vi "puls_generator_control.VI"() -> ()   [LabVIEW 2015]
uses:
  board.vis/Globals.vi
panel:
  in  "TM0H":u16
  in  "TM0L":u16=1000
  in  "DO8":u16
  in  "TO8":u16
  in  "DO7":u16
  in  "TO7":u16
  in  "DO6":u16
  in  "TO6":u16
  in  "DO5":u16
  in  "TO5":u16
  in  "DO4":u16
  in  "T04":u16
  in  "DO3":u16
  in  "TO3":u16
  in  "D02":u16=100
  in  "TO2":u16=10
  in  "Send O CTRL":bool
  out "cams recognised":u8=2
  # "Tn: delay"
  # "Dn: duration"
  # "*5ns"
  # "TO1: T0 main clock"
  # "period"
  # "*10ns"
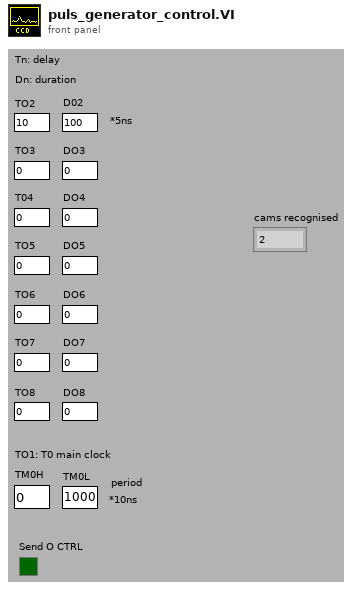
[diagram p1: front panel]
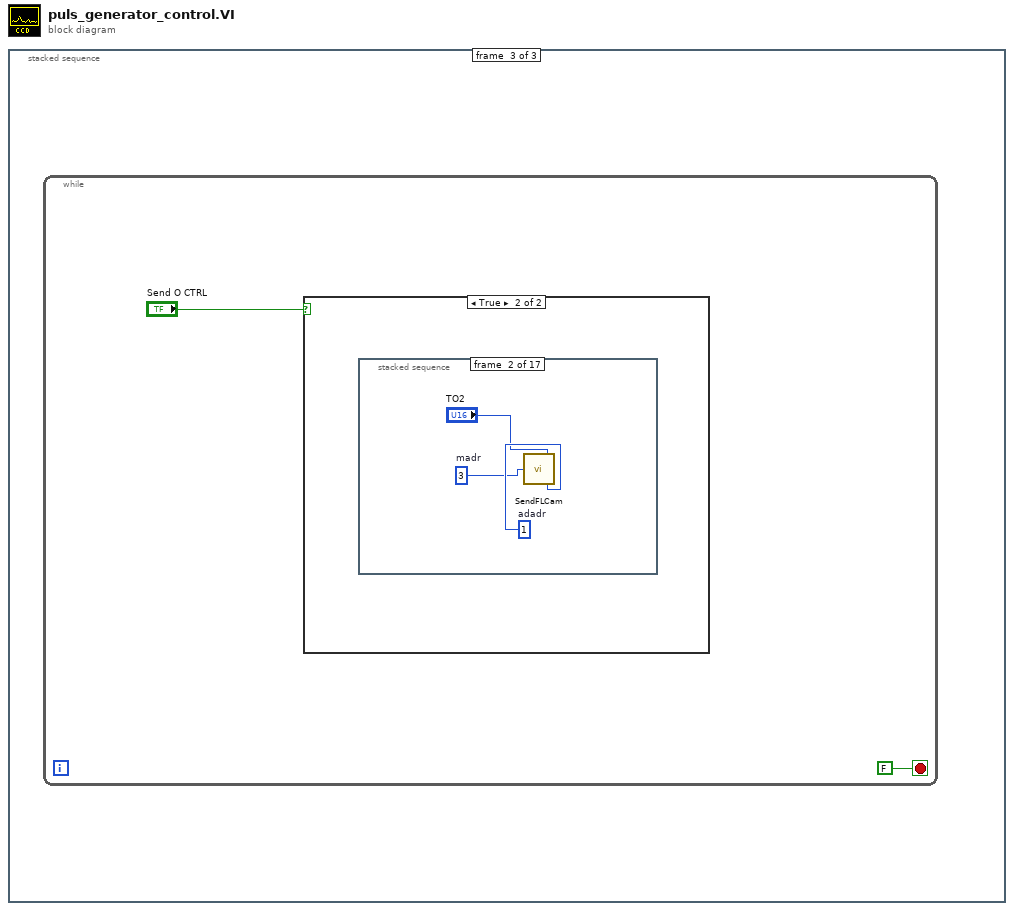
[diagram p0: block diagram]
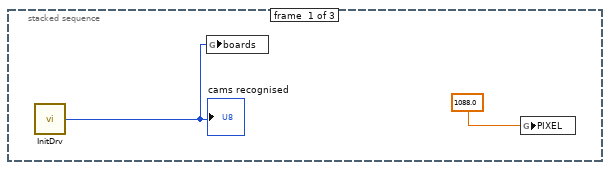
[diagram p2: hidden frame]
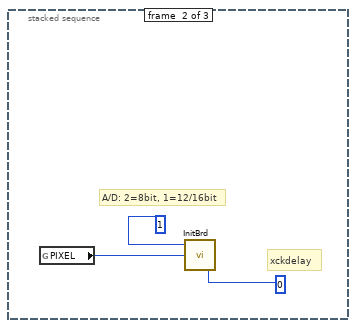
[diagram p3: hidden frame]
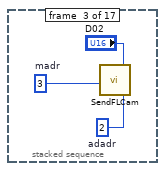
[diagram p6: hidden frame]
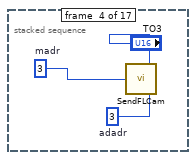
[diagram p7: hidden frame]
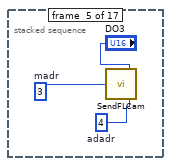
[diagram p8: hidden frame]
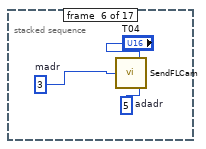
[diagram p9: hidden frame]
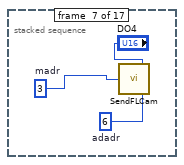
[diagram p10: hidden frame]
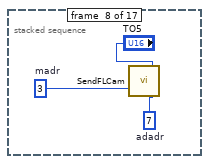
[diagram p11: hidden frame]
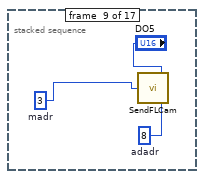
[diagram p12: hidden frame]
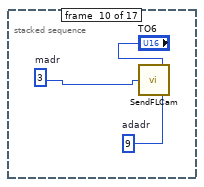
[diagram p13: hidden frame]
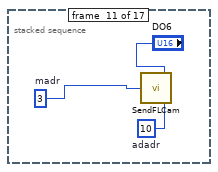
[diagram p14: hidden frame]
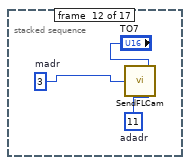
[diagram p15: hidden frame]
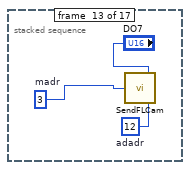
[diagram p16: hidden frame]
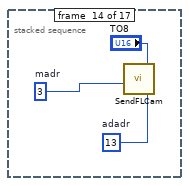
[diagram p17: hidden frame]
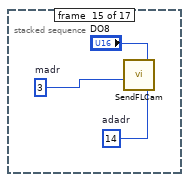
[diagram p18: hidden frame]
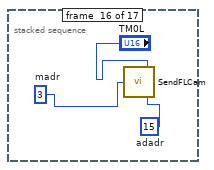
[diagram p19: hidden frame]
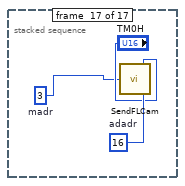
[diagram p20: hidden frame]
diagram:
  n1 = stacked-sequence {
    frame #0 {
      n2 = call "InitDrv.vi"() -> ("Boards"=w2:u8)  [unwired: 1 in]
      "cams recognised" <- w2
      n3 = global write "Globals.vi" "boards"(w2) -> ()
      n4 = global write "Globals.vi" "PIXEL"(1088.0) -> ()
    }
    frame #1 {
      # "xckdelay"
      # "A/D: 2=8bit, 1=12/16bit"
      n5 = global read "Globals.vi" "PIXEL"() -> (w3:u32)
      n6 = call "InitBrd.vi"("xckdly"=u32 0, "pixel"=w3, "flag816"=u32 1) -> ()  [unwired: 3 in]
    }
    frame #2 {
      n7 = while {
        stop <- FALSE stop-if-true
        n8 = case shown="True" "Send O CTRL" {
          frame False {
          }
          frame True {
            n9 = stacked-sequence {
              frame #0 {
              }
              frame #1 {
                w10 = 1  # adadr
                w9 = 3  # madr
                n10 = call "SendFLCam.vi"("madr"=w9, "data"="TO2", "adadr"=w10) -> ()
              }
              frame #2 {
                w12 = 2  # adadr
                w13 = 3  # madr
                n11 = call "SendFLCam.vi"("madr"=w13, "data"="D02", "adadr"=w12) -> ()
              }
              frame #3 {
                w16 = 3  # adadr
                w15 = 3  # madr
                n12 = call "SendFLCam.vi"("madr"=w15, "data"="TO3", "adadr"=w16) -> ()
              }
              frame #4 {
                w19 = 4  # adadr
                w18 = 3  # madr
                n13 = call "SendFLCam.vi"("madr"=w18, "data"="DO3", "adadr"=w19) -> ()
              }
              frame #5 {
                w22 = 5  # adadr
                w21 = 3  # madr
                n14 = call "SendFLCam.vi"("madr"=w21, "data"="T04", "adadr"=w22) -> ()
              }
              frame #6 {
                w25 = 6  # adadr
                w24 = 3  # madr
                n15 = call "SendFLCam.vi"("madr"=w24, "data"="DO4", "adadr"=w25) -> ()
              }
              frame #7 {
                w28 = 7  # adadr
                w27 = 3  # madr
                n16 = call "SendFLCam.vi"("madr"=w27, "data"="TO5", "adadr"=w28) -> ()
              }
              frame #8 {
                w31 = 8  # adadr
                w30 = 3  # madr
                n17 = call "SendFLCam.vi"("madr"=w30, "data"="DO5", "adadr"=w31) -> ()
              }
              frame #9 {
                w32 = 9  # adadr
                w34 = 3  # madr
                n18 = call "SendFLCam.vi"("madr"=w34, "data"="TO6", "adadr"=w32) -> ()
              }
              frame #10 {
                w37 = 10  # adadr
                w36 = 3  # madr
                n19 = call "SendFLCam.vi"("madr"=w36, "data"="DO6", "adadr"=w37) -> ()
              }
              frame #11 {
                w40 = 11  # adadr
                w39 = 3  # madr
                n20 = call "SendFLCam.vi"("madr"=w39, "data"="TO7", "adadr"=w40) -> ()
              }
              frame #12 {
                w43 = 12  # adadr
                w42 = 3  # madr
                n21 = call "SendFLCam.vi"("madr"=w42, "data"="DO7", "adadr"=w43) -> ()
              }
              frame #13 {
                w45 = 13  # adadr
                w46 = 3  # madr
                n22 = call "SendFLCam.vi"("madr"=w46, "data"="TO8", "adadr"=w45) -> ()
              }
              frame #14 {
                w48 = 14  # adadr
                w49 = 3  # madr
                n23 = call "SendFLCam.vi"("madr"=w49, "data"="DO8", "adadr"=w48) -> ()
              }
              frame #15 {
                w51 = 15  # adadr
                w52 = 3  # madr
                n24 = call "SendFLCam.vi"("madr"=w52, "data"="TM0L", "adadr"=w51) -> ()
              }
              frame #16 {
                w55 = 16  # adadr
                w53 = 3  # madr
                n25 = call "SendFLCam.vi"("madr"=w53, "data"="TM0H", "adadr"=w55) -> ()
              }
            }
          }
        }
      }
    }
  }
